vi "Clean Filename.vi"(6 "Clean Filename?":bool, 11 "Filepath in":path) -> (2 "Filename out":string, 3 "Filepath out":path)   [LabVIEW 2024]
uses:
  <vilib>/Utility/error.llb/Trim Whitespace One-Sided.vi
  <userlib>/_OpenG.lib/file/file.llb/Strip Path Extension - String__ogtk.vi
  <vilib>/regexp/Match Regular Expression.xnode
  <userlib>/_OpenG.lib/file/file.llb/openg_file.lvlib
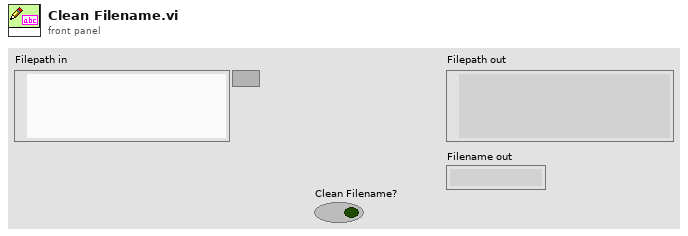
[diagram p1: front panel]
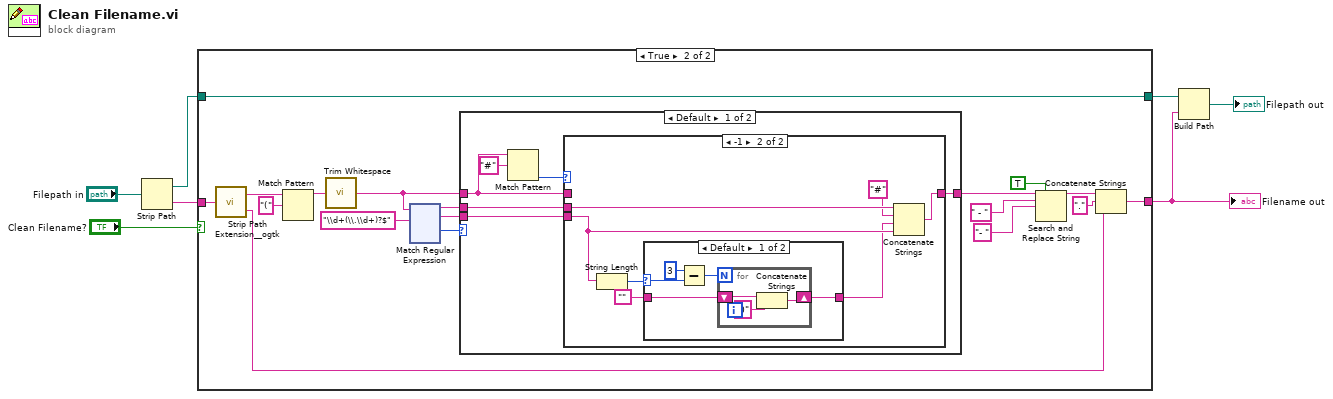
[diagram p0: block diagram]
diagram:
  n1 = Strip Path(path="Filepath in") -> (stripped path=w5:path, name=w4:string)
  n2 = case shown="True" "Clean Filename?" {
    tunnel: [w9 w10] -> w3
    tunnel: [w8 w12] -> w2
    tunnel: w5 -> [w9 w10]
    tunnel: w4 -> [w8 w11]
    frame False {
    }
    frame True {
      n3 = call-poly <userlib>:"Strip Path Extension__ogtk.vi"("path"=w11) -> ("root"=w27:string, "extension"=w24:string)
      n4 = Match Pattern(string=w27, regular expression="(") -> (before substring=w25:string)  [unwired: 1 in, 3 out]
      n5 = call <vilib>:"Trim Whitespace.vi"("string"=w25) -> ("trimmed string"=w15:string)  [unwired: 1 in]
      n6 = xnode "Match Regular Expression"("input string"=w15, "regular expression"="\\d+(\\.\\d+)?$") -> ("before match"=w14:string, "whole match"=w13:string, "offset past match"=w18:i32)  [unwired: 4 in, 2 out]
      n7 = case shown="Default" w18 {
        tunnel: [w32 w51] -> w16
        tunnel: w15 -> [w30 w51]
        tunnel: w14 -> [w33 _]
        tunnel: w13 -> [w31 _]
        frame Default {
          n8 = Match Pattern(string=w30, regular expression="#") -> (offset past match=w28:i32)  [unwired: 1 in, 3 out]
          n9 = case shown="-1" w28 {
            tunnel: w33 -> [_ w41]
            tunnel: [w34 w39] -> w32
            tunnel: w31 -> [_ w37]
            tunnel: w30 -> [w34 _]
            frame Default {
            }
            frame -1 {
              n10 = String Length(string=w37) -> (length=w38:i32)
              n11 = case shown="Default" w38 {
                selector: w38 -> [w46 _]
                tunnel: [w43 w50] -> w36
                tunnel: "" -> [w42 w50]
                frame Default {
                  n12 = Subtract(x=3, y=w46) -> (x-y=w44:i32)
                  n13 = for {
                    N: w44 -> [_]
                    shift-right: [w49] -> w43
                    shift-left: w42 -> [w48]
                    n14 = Concatenate Strings(w48, "0" ("string")) -> (w49:string)
                  }
                }
                frame 3.. {
                }
              }
              n15 = Concatenate Strings(w41, "#", w36, w37) -> (w39:string)
            }
          }
        }
        frame -1 {
        }
      }
      n16 = Search and Replace String(replace all?=TRUE ("replace all? (F)"), input string=w16, search string=" - " ("string"), replace string="- " ("string")) -> (result string=w22:string)  [unwired: 4 in, 3 out]
      n17 = Concatenate Strings(w22, "." ("string"), w24) -> (w12:string)
    }
  }
  "Filename out" <- w2
  n18 = Build Path(base path=w3, name or relative path=w2) -> (appended path=→"Filepath out":path)
